vi "Save_Info.vi"(8 "error in (no error)":errorcluster, 11 "AB_EXE in":refnum<class "AB_EXE.lvclass">) -> (0 "error out":errorcluster, 3 "AB_EXE out":refnum<class "AB_EXE.lvclass">)   [LabVIEW 2020, in "AB_EXE.lvclass"]
uses:
  <vilib>/AppBuilder/AB_Classes/EXE/AB_EXE.lvclass
  e:/builds/penguin/labview/branches/2020/dev/dist/vi.lib/AppBuilder/AB_Classes/Build/AB_Build.lvclass
  <vilib>/AppBuilder/RW_Project/AB_RW_Project_EXE_SharedVar_Deploy.ctl
  <vilib>/AppBuilder/RW_Project/AB_RW_Project_EXE_SharedVar_LibInfo.ctl
  <vilib>/AppBuilder/RW_Project/AB_RW_Project_EXE_Data.ctl
  <vilib>/AppBuilder/RW_Project/AB_RW_Project_PropBag_Action.ctl
  <vilib>/AppBuilder/AB_Classes/EXE/AB_EXE.lvclass/AB_EXE.ctl
  <vilib>/AppBuilder/AB_Classes/Application/AB_Application.lvclass
  <vilib>/AppBuilder/AB_Classes/Build/AB_Build.lvclass
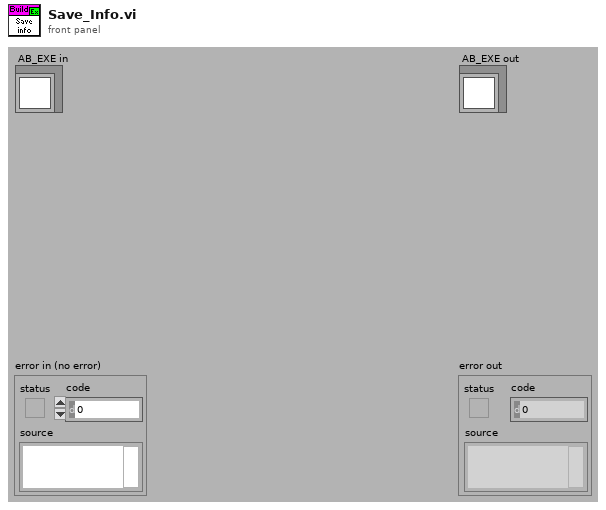
[diagram p1: front panel]
types:
  T1 = typedef "AB_RW_Project_EXE_SharedVar_Deploy.ctl" = cluster{"deploy at startup":bool, "undeploy on exit":bool, "variable libraries":T2[], "hide deployment dialog":bool}
  T2 = typedef "AB_RW_Project_EXE_SharedVar_LibInfo.ctl" = cluster{"LibraryItemID":string, "deploy":bool}
  T3 = typedef "AB_RW_Project_EXE_Data.ctl" = cluster{"cmdLineArgs":bool, "actXServerName":string, "actXServerNameGUID":string, "iconItemID":string, "var deploy data":T1}
  T4 = typedef "AB_RW_Project_PropBag_Action.ctl" = enum16{"read", "write", "clear", "readPrevious", "writePrevious", "clearPrevious"}
  T5 = typedef "AB_EXE_SharedVar_Deploy.ctl" = cluster{"deploy at startup":bool, "undeploy on exit":bool, "variable libraries":T6[], "hide deployment dialog":bool}
  T6 = typedef "AB_EXE_SharedVar_LibInfo.ctl" = cluster{"LibraryPath":path, "LibraryItemID":string, "target":string, "deploy":bool}
  T7 = typedef "AB_Build.ctl" = cluster{"buildSpecName":string, "buildSpecDescription":string, "destinations":refnum<class "AB_Destination.lvclass">[], "exclusionOption":T8, "defaultLanguage":string, "supportedLanguages":string[], "excludedDirectories":path[], "buildContext":refnum<vi>, "buildObject":T9, "preview":bool, "programatic":bool, "progressBarEvents":T10, "userLog_Path":path, "preActionID":string, "preAction_Path":path, "postActionID":string, "postAction_Path":path, "eng_checkForBrokenVIs?":bool, "eng_verboseLinkerErrors?":bool, "localDest_Path":path, "targetDest_Path":path, "removeVIObject":u16, "cache":refnum<class "PreviewCache.lvclass">, "use cache":bool, "previewCache_ID":string, "buildCache_ID":string, "eng_TempLocalDest_Path":path, "eng_collectDependencies?":bool, "versionInfo":cluster{"buildVersion":cluster{"major":u16, "minor":u16, "patch":u16, "build":u16}, "autoIncrement":bool}, "eng_enableVIChecksums":bool}
  T8 = typedef "AB_Exclusion_Option.ctl" = cluster{"typedefs":bool, "polymorphicVIs":bool, "unusedLibraryItems":bool, "modifyLibraryFile":bool, "edit-timeDependencies":bool, "inlineVIs":bool, "dependent PPLs":bool, "dependent DLLs":bool}
  T9 = typedef "ItemRef.ctl" = u64
  T10 = typedef "provcom_ProgressBar_Events.ctl" = cluster{"newJob":refnum<user-event>, "newItem":refnum<user-event>, "errorMsg":T11, "cancel":refnum<user-event>}
  T11 = typedef "mxLvBuildError.ctl" = refnum<user-event>
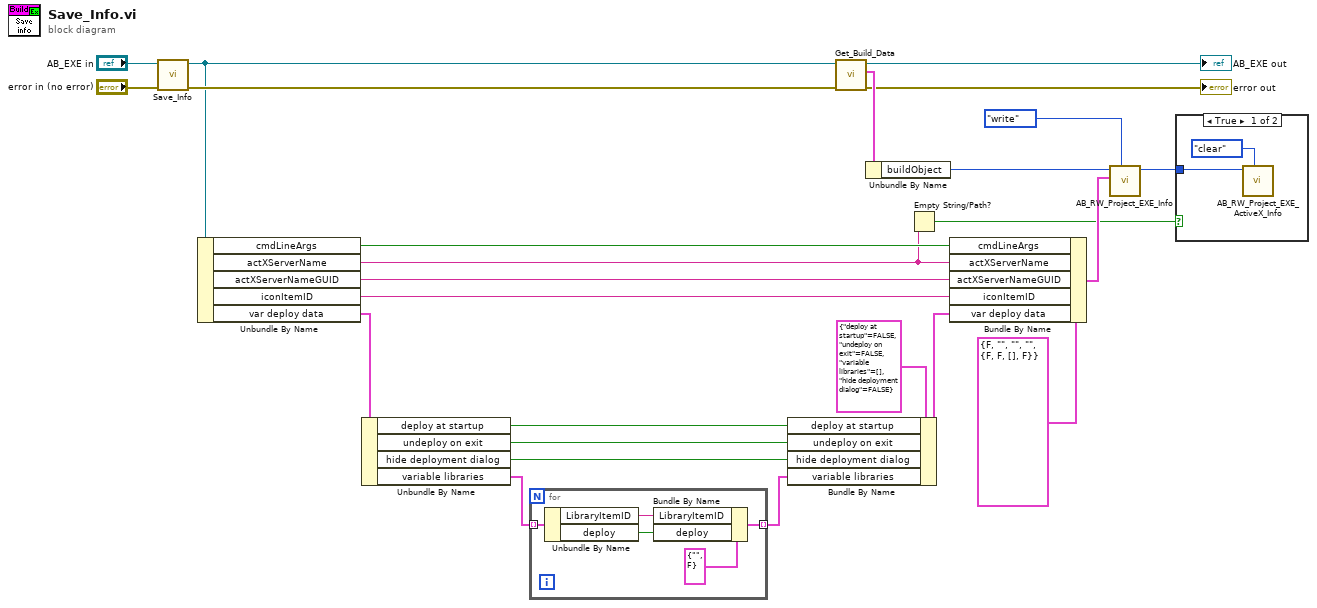
[diagram p0: block diagram]
diagram:
  n1 = call-parent "Save_Info.vi"("error in (no error)"="error in (no error)", "AB_Application in"="AB_EXE in") -> ("error out"=w14:errorcluster, "AB_Application out"=w12:refnum<class "AB_EXE.lvclass">)  [unwired: 8 out]
  n2 = Unbundle By Name(w12) -> ("cmdLineArgs"=w21:bool, "actXServerName"=w16:string, "actXServerNameGUID"=w11:string, "iconItemID"=w19:string, "var deploy data"=w9:T5)
  n3 = Unbundle By Name(w9) -> ("deploy at startup"=w7:bool, "undeploy on exit"=w6:bool, "hide deployment dialog"=w2:bool, "variable libraries"=w4:T6[])
  n4 = for {
    tunnel: w4 -> [w30] mode=indexing
    tunnel: [w26] -> w3 mode=indexing
    n5 = Unbundle By Name(w30) -> ("LibraryItemID"=w28:string, "deploy"=w27:bool)
    n6 = Bundle By Name(cluster=T2 {"LibraryItemID"="", "deploy"=FALSE} ("variable libraries"), "LibraryItemID"=w28, "deploy"=w27) -> (w26:T2)
  }
  n7 = Bundle By Name(cluster=T1 {"deploy at startup"=FALSE, "undeploy on exit"=FALSE, "variable libraries"=[], "hide deployment dialog"=FALSE} ("var deploy data"), "deploy at startup"=w7, "undeploy on exit"=w6, "hide deployment dialog"=w2, "variable libraries"=w3) -> (w5:T1)
  n8 = call <vilib>:"Get_Build_Data.vi"("error in (no error)"=w14, "Class in"=w12) -> ("error out"=→"error out":errorcluster, "data"=w15:T7, "Class out"=→"AB_EXE out":refnum<class "AB_EXE.lvclass">)  [unwired: 7 out]
  n9 = Unbundle By Name(w15) -> ("buildObject"=w1:T9)
  n10 = Empty String/Path?(string/path=w16) -> (empty?=w18:bool)
  n11 = Bundle By Name(cluster=T3 {"cmdLineArgs"=FALSE, "actXServerName"="", "actXServerNameGUID"="", "iconItemID"="", "var deploy data"={"deploy at startup"=FALSE, "undeploy on exit"=FALSE, "variable libraries"=[], "hide deployment dialog"=FALSE}} ("Exe_info in"), "cmdLineArgs"=w21, "actXServerName"=w16, "actXServerNameGUID"=w11, "iconItemID"=w19, "var deploy data"=w5) -> (w20:T3)
  n12 = call <vilib>:"AB_RW_Project_EXE_Info.vi"("action"=AB_RW_Project_PropBag_Action."write", "Exe_info in"=w20, "Object In"=w1) -> ("Object Out"=w17:T9)  [unwired: 1 in, 7 out]
  n13 = case shown="True" w18 {
    tunnel: w17 -> [w31 _]
    frame True {
      n14 = call <vilib>:"AB_RW_Project_EXE_ActiveX_Info.vi"("action"=AB_RW_Project_PropBag_Action."clear", "Object In"=w31) -> ()  [unwired: 2 in, 8 out]
    }
    frame False {
    }
  }
